vi "Points.vi"(6 "Количество точек":dbl, 9 "Частота (1000 Hz)":dbl, 10 "Ширина импульса, тчк":dbl=1000.0, 11 "Точек между импульсами, тчк":dbl) -> (0 "Детектор":i32[](array[numeric]), 2 "Количество точек":string caption="String", 3 "Начало второго импульса":string, 4 "Диод":i32[](array[numeric]), 5 "Оставшиеся точки":string, 7 "Начало интервала":string)   [LabVIEW 2012]
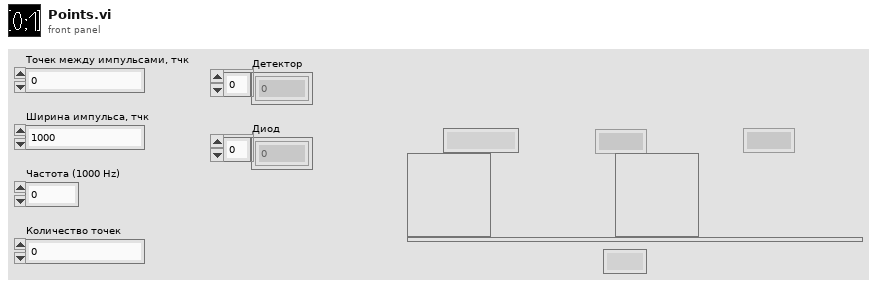
[diagram p1: front panel]
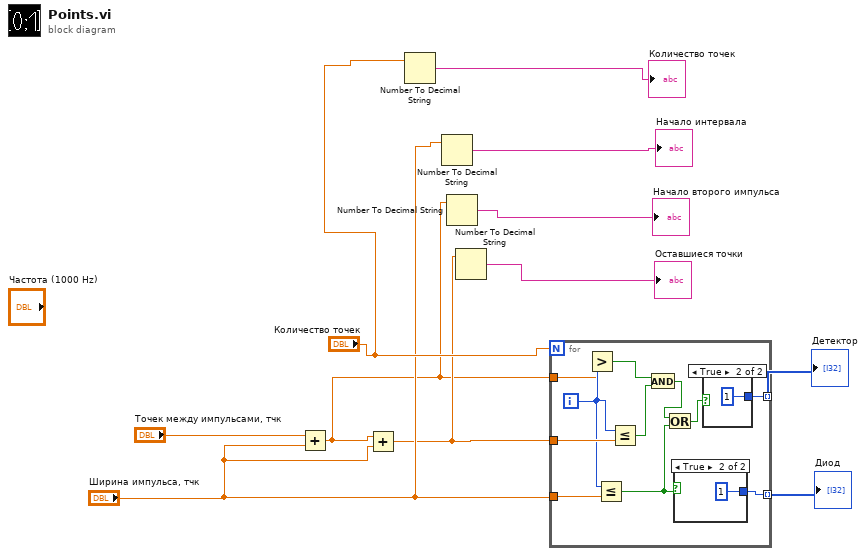
[diagram p0: block diagram]
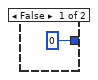
[diagram p2: hidden frame]
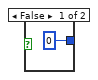
[diagram p3: hidden frame]
diagram:
  n1 = Add(x="Точек между импульсами, тчк", y="Ширина импульса, тчк") -> (x+y=w1:dbl)
  n2 = Add(x=w1, y="Ширина импульса, тчк") -> (x+y=w2:dbl)
  n3 = Number To Decimal String(number="Количество точек") -> (decimal integer string=→"Количество точек":string)  [unwired: 1 in]
  n4 = Number To Decimal String(number="Ширина импульса, тчк") -> (decimal integer string=→"Начало интервала":string)  [unwired: 1 in]
  n5 = Number To Decimal String(number=w1) -> (decimal integer string=→"Начало второго импульса":string)  [unwired: 1 in]
  n6 = Number To Decimal String(number=w2) -> (decimal integer string=→"Оставшиеся точки":string)  [unwired: 1 in]
  n7 = for {
    N: "Количество точек" -> [_]
    tunnel: [w22] -> w6 mode=indexing
    tunnel: "Ширина импульса, тчк" -> [w21]
    tunnel: w1 -> [w17]
    tunnel: w2 -> [w20]
    tunnel: [w19] -> w7 mode=indexing
    i -> [w18]
    n8 = Greater?(x=w18, y=w17) -> (0:w16:bool)
    n9 = Less Or Equal?(x=w18, y=w21) -> (x <= y?=w12:bool)
    n10 = Less Or Equal?(x=w18, y=w20) -> (x <= y?=w15:bool)
    n11 = And(x=w16, y=w15) -> (x .and. y?=w14:bool)
    n12 = Or(x=w14, y=w12) -> (x .or. y?=w13:bool)
    n13 = case shown="True" w12 {
      tunnel: [0 1] -> w19
      frame False {
      }
      frame True {
      }
    }
    n14 = case shown="True" w13 {
      tunnel: [0 1] -> w22
      frame False {
      }
      frame True {
      }
    }
  }
  "Диод" <- w7
  "Детектор" <- w6
